vi "Night.vi"(10 "Do":i32, 11 "Od":i32) -> (3 "Noc":bool)   [LabVIEW 2014]
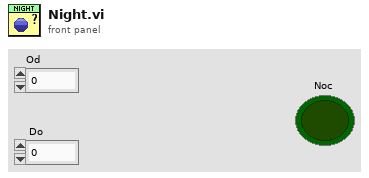
[diagram p1: front panel]
types:
  T1 = typedef "LVDateTimeRec.ctl" = cluster{"fractional second":dbl, "second":i32, "minute":i32, "hour":i32, "day of month":i32, "month":i32, "year":i32, "day of week":i32, "day of year":i32, "DST":i32}
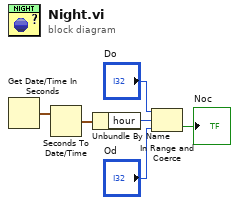
[diagram p0: block diagram]
diagram:
  n1 = Get Date/Time In Seconds() -> (seconds since 1Jan1904=w6:timestamp)
  n2 = Seconds To Date/Time(time stamp (now)=w6) -> (date time rec=w5:T1)  [unwired: 1 in]
  n3 = Unbundle By Name(w5) -> ("hour"=w4:i32)
  n4 = In Range and Coerce(upper limit="Do", x=w4, lower limit="Od") -> (In Range?=→"Noc":bool)  [unwired: 1 out]
